vi "Timed Read from Hardware.vi"(8 "error in":errorcluster, 10 "values":dbl[](array[numeric]), 11 "execution unit":refnum<class "Execution Unit.lvclass">) -> (0 "error out":errorcluster, 2 "values out":dbl[](array[numeric]), 3 "execution unit out":refnum<class "Execution Unit.lvclass">)   [LabVIEW 2020, in "AIM MIL-STD-1553 Engine.lvlib" / "Custom Device.lvlib"]
uses:
  Custom Device.lvlib
  Interfaces/Execution Unit/Execution Unit.lvclass
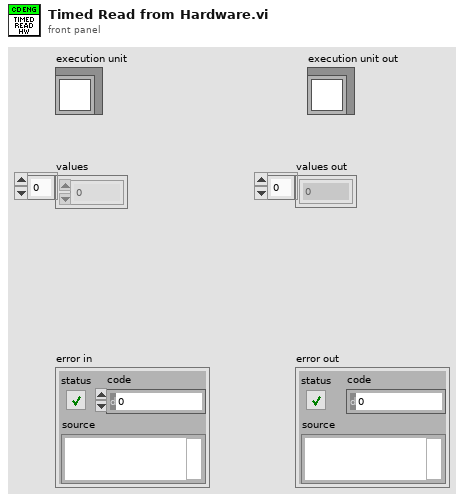
[diagram p1: front panel]
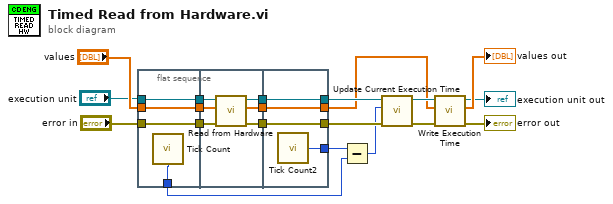
[diagram p0: block diagram]
diagram:
  n1 = flat-sequence {
    tunnel: "values" -> [w22]
    tunnel: "error in" -> [w23]
    tunnel: "execution unit" -> [w24]
    tunnel: [w24] -> w20
    tunnel: [w23] -> w19
    tunnel: [w22] -> w18
    tunnel: [w21] -> w14
    tunnel: w20 -> [w28]
    tunnel: w19 -> [w27]
    tunnel: w18 -> [w26]
    tunnel: [w30] -> w17
    tunnel: [w29] -> w16
    tunnel: [w25] -> w15
    tunnel: [w32] -> w3
    tunnel: [w33] -> w7
    tunnel: [w34] -> w8
    tunnel: w17 -> [w34]
    tunnel: w16 -> [w33]
    tunnel: w15 -> [w32]
    tunnel: [w31] -> w13
    frame #0 {
      n2 = call "Tick Count"() -> ("Tick Count(uSec)"=w21:u32)
    }
    frame #1 {
      n3 = call-dynamic "Read from Hardware.vi"("error in (no error)"=w27, "Values in"=w26, "Execution Unit in"=w28) -> ("error out"=w30:errorcluster, "Values out"=w25:dbl[], "Execution Unit out"=w29:refnum<class "Execution Unit.lvclass">)  [unwired: 6 in]
    }
    frame #2 {
      n4 = call "Tick Count2"() -> ("Tick Count(uSec)"=w31:u32)
    }
  }
  n5 = Subtract(x=w13, y=w14) -> (x-y=w6:u32)
  n6 = call-dynamic "Update Current Execution Time.vi"("error in (no error)"=w8, "Current Execution Time (us)"=w6, "Execution Unit in"=w7) -> ("error out"=w5:errorcluster, "Execution Unit out"=w4:refnum<class "Execution Unit.lvclass">)  [unwired: 7 in]
  n7 = call-dynamic "Write Execution Time.vi"("error in (no error)"=w5, "Values in"=w3, "Execution Unit in"=w4) -> ("error out"=→"error out":errorcluster, "Values out"=→"values out":dbl[], "Execution Unit out"=→"execution unit out":refnum<class "Execution Unit.lvclass">)  [unwired: 6 in]
